vi "TLV Parser.vi"() -> ()   [LabVIEW 2017]
panel:
  out "Array 2":string[](array[string])
  out "Array":T1(array[cluster]) {"Value" format="%.0x"}
  in  "Threshold":dbl format="%#_13g"
  in  "file (use dialog)":path
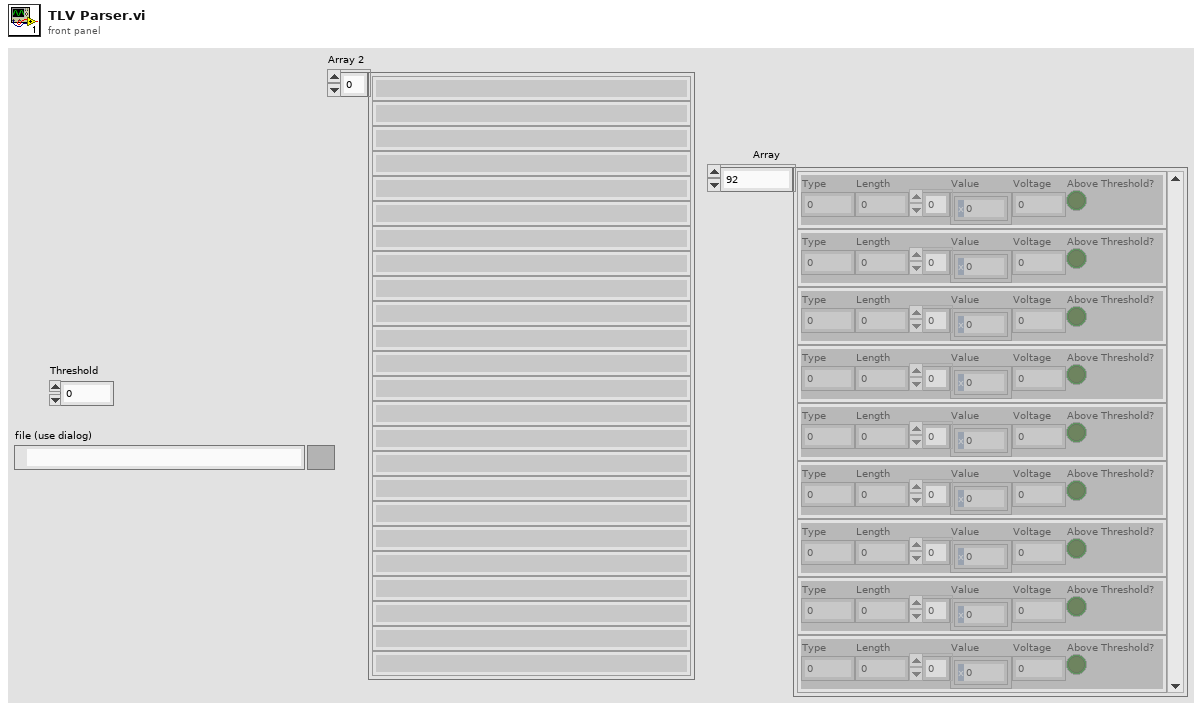
[diagram p1: front panel]
types:
  T1 = cluster{"Type":u8, "Length":u8, "Value":u8[], "Voltage":dbl, "Above Threshold?":bool}[]
  T2 = enum16{"open", "replace", "create", "open or create", "replace or create", "replace or create with confirmation"}
  T3 = cluster{"Type":u8, "Length":u8, "Value":u8[], "Voltage":dbl, "Above Threshold?":bool}
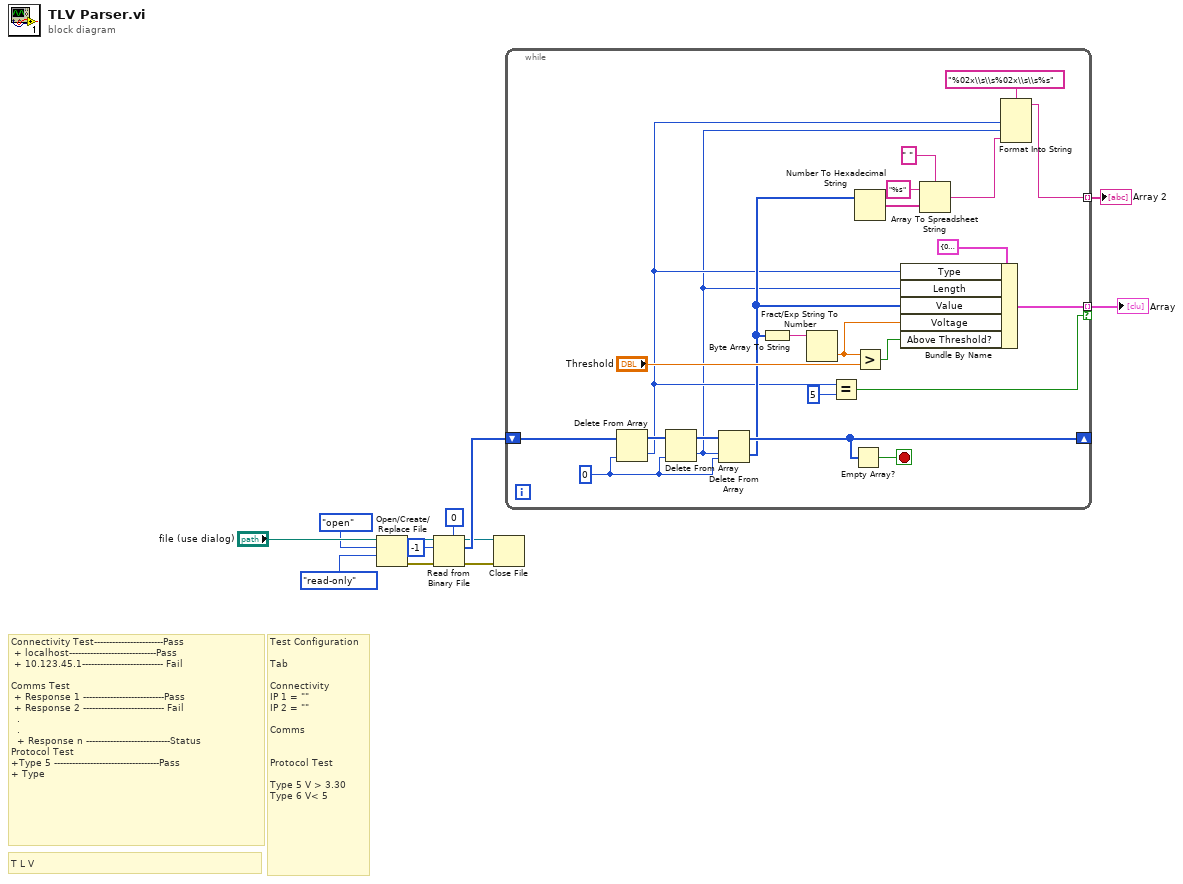
[diagram p0: block diagram]
diagram:
  # "T L V"
  # "Test Configuration\n\nTab\n\nConnectivity\nIP 1 = \"\"\nIP 2 = \"\"\n\nComms\n\n\nProtocol Test\n\nType 5 V > 3.30\nType 6 V< 5"
  # "Connectivity Test-----------------------Pass\n + localhost-----------------------------Pass\n + 10.123.45.1--------------------------- Fail\n\nComms Test\n + Response 1 ---------------------------Pass\n + Response 2 --------------------------- Fail\n  .\n  .\n  + Response n ----------------------------Status\nProtocol Test\n+Type 5 -----------------------------------Pass\n+ Type"
  n1 = Open/Create/Replace File(file path (use dialog)="file (use dialog)", operation (0:open)=T2."open", access (0:read/write)=enum16{"read/write", "read-only", "write-only"}."read-only") -> (refnum out=w7:refnum<file>, error out=w6:errorcluster)  [unwired: 3 in, 1 out]
  n2 = Read from Binary File(5:u8 0 ("Numeric"), 8:w6, 10:-1 ("count (1)"), 11:w7) -> (0:w2:errorcluster, 2:w10:u8[], 3:w3:refnum<file>)  [unwired: 2 in, 1 out]
  n3 = Close File(refnum=w3, error in=w2) -> ()  [unwired: 2 out]
  n4 = while {
    shift-right: [w29] -> _
    shift-left: w10 -> [w32]
    tunnel: [w35] -> w9 mode=indexing if=w13
    tunnel: [w14] -> w1 mode=indexing
    stop <- w33 stop-if-true
    w28 = 0 ("index")
    n5 = Delete From Array(array=w32, index=w28) -> (deleted portion=w17:u8, array with subset deleted=w31:u8[])  [unwired: 1 in]
    n6 = Delete From Array(array=w31, index=w28) -> (deleted portion=w16:u8, array with subset deleted=w30:u8[])  [unwired: 1 in]
    n7 = Delete From Array(array=w30, length=w16, index=w28) -> (deleted portion=w19:u8[], array with subset deleted=w29:u8[])
    n8 = Byte Array To String(unsigned byte array=w19) -> (string=w26:string)
    n9 = Fract/Exp String To Number(string=w26) -> (number=w25:dbl)  [unwired: 3 in, 1 out]
    n10 = Equal?(x=w17, y=u8 5) -> (x = y?=w13:bool)
    n11 = Empty Array?(array=w29) -> (empty?=w33:bool)
    n12 = Number To Hexadecimal String(2:w19) -> (0:w22:string[])  [unwired: 1 in]
    n13 = Greater?(x=w25, y="Threshold") -> (0:w23:bool)
    n14 = Bundle By Name(cluster=T3 {"Type"=0, "Length"=0, "Value"=[], "Voltage"=0.0, "Above Threshold?"=TRUE}, "Type"=w17, "Length"=w16, "Value"=w19, "Voltage"=w25, "Above Threshold?"=w23) -> (w35:T3)
    n15 = Array To Spreadsheet String(delimiter (Tab)=" ", array=w22, 3:"%s" ("format string")) -> (spreadsheet string=w15:string)
    n16 = Format Into String(format string="%02x\\s\\s%02x\\s\\s%s", w17, w16, w15) -> (resulting string=w14:string)  [unwired: 2 in, 1 out]
  }
  "Array" <- w9
  "Array 2" <- w1
